vi "kb-Point22.vi"(10 "Src Data":dbl[][](array[numeric]), 11 "ROI Descriptor":T1 {"Contours"."Type" items=["No Selection", "Point", "Line", "Rectangle", "Oval", "Polygon", "Freehand Region", "Annulus", "Unused2", "Unused3", "Broken Line", "Freehand Line", "Rotated Rectangle"]}) -> ()   [LabVIEW 2015]
uses:
  <vilib>/Math Plots/3D Math Plots/3D Surface/3D Surface XCtrl/3D Surface.xctl
  <vilib>/Math Plots/3D Math Plots/3D Surface/3D Surface Datatype/Public/Plot Helper (Matrix).vi
  <vilib>/Math Plots/3D Math Plots/3D Surface/3D Surface Datatype/3D Surface Datatype.lvclass
panel:
  out "3D Surface 3":refnum<class "3D Plot Datatype.lvclass">[](xcontrol) caption="三维曲面"
  out "最大值":dbl
  out "3D Surface 2":refnum<class "3D Plot Datatype.lvclass">[](xcontrol) caption="三维曲面"
  out "3D Surface":refnum<class "3D Plot Datatype.lvclass">[](xcontrol) caption="三维曲面"
  out "Coordinates 2":i32[](array[numeric])
  out "Radius (Pixels)":dbl
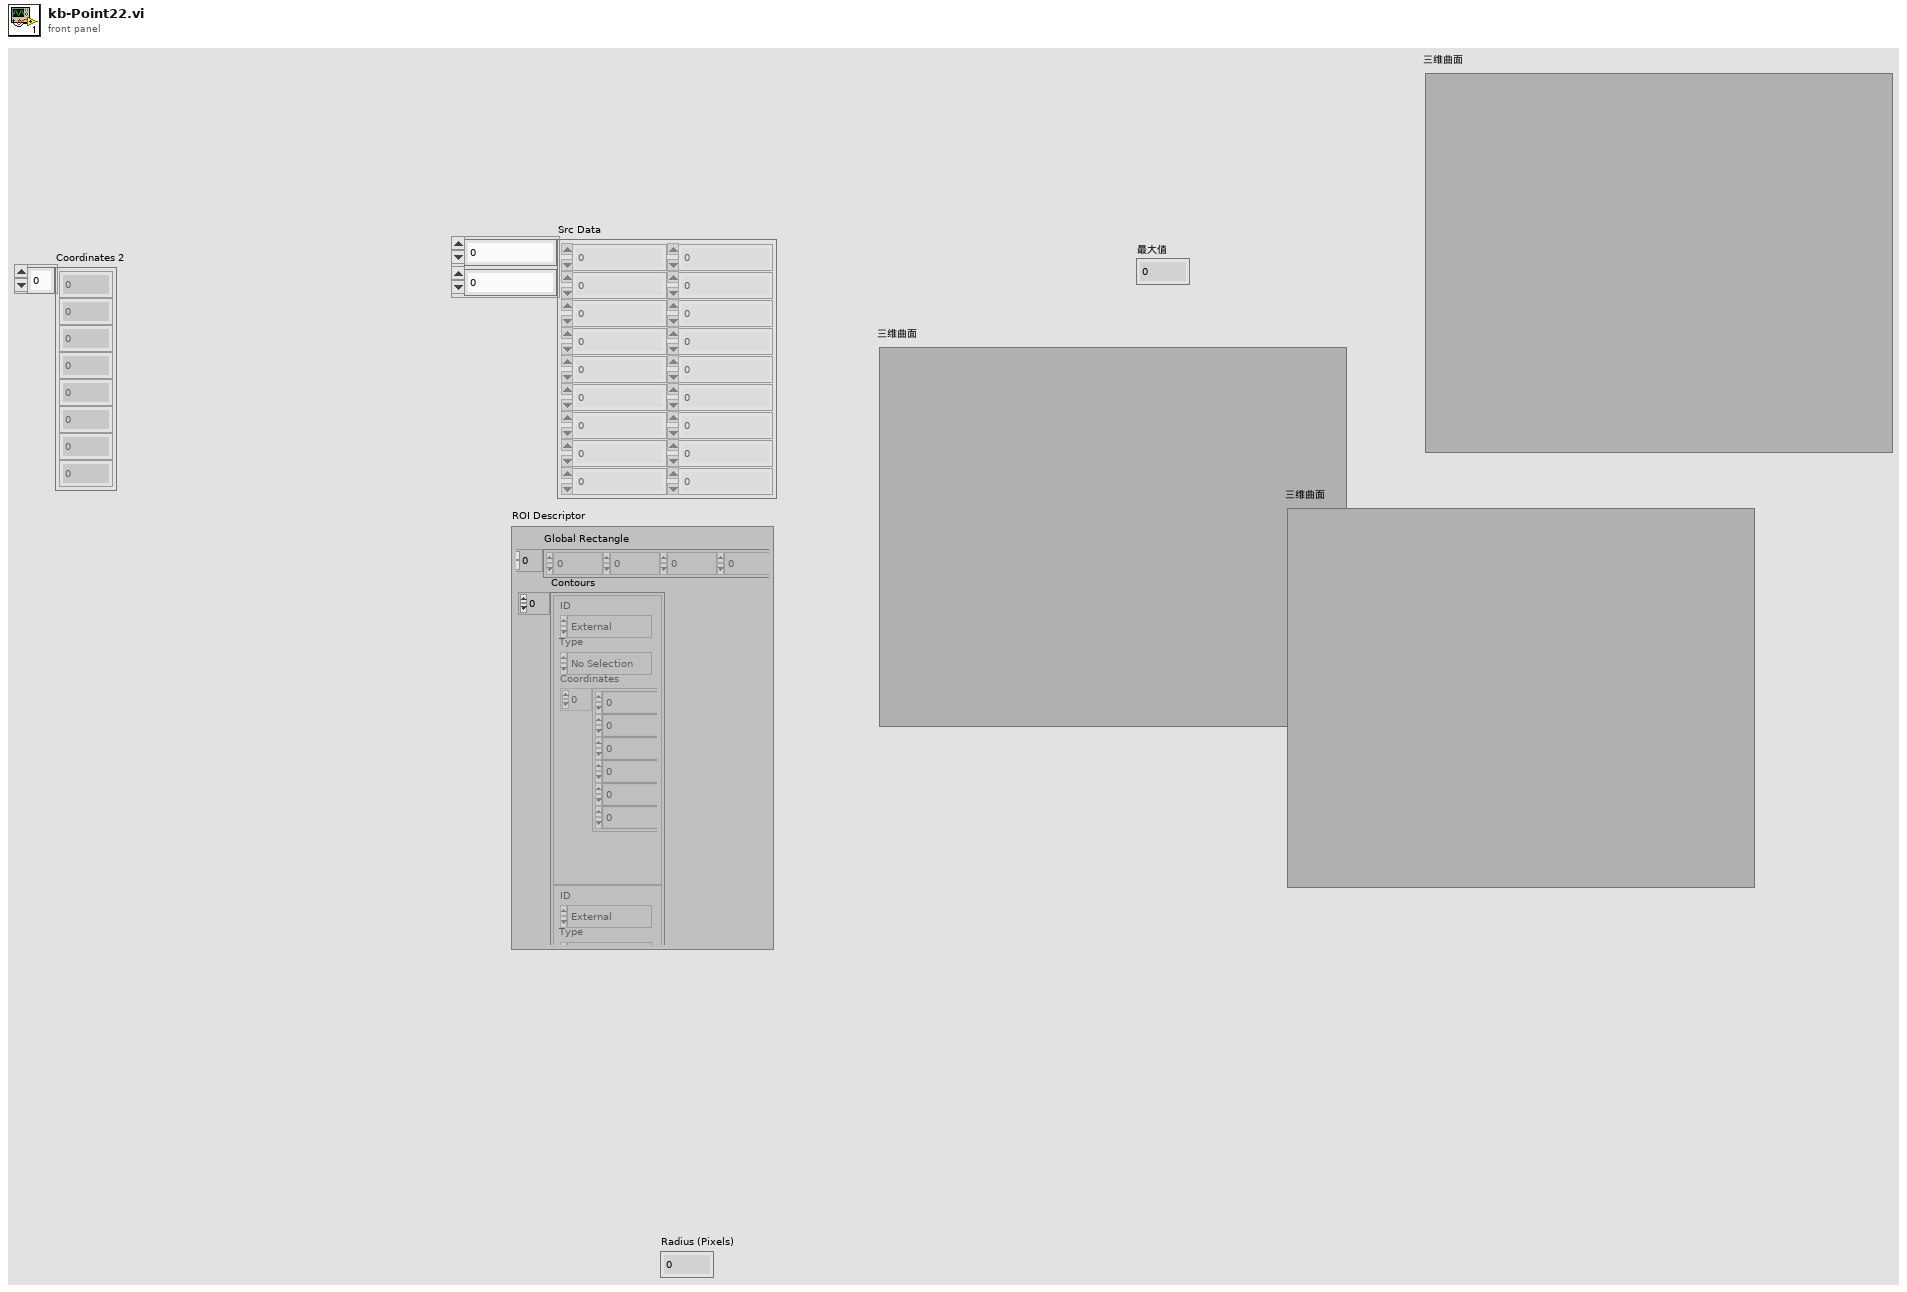
[diagram p1: front panel]
types:
  T1 = typedef "ROI Descriptor" = cluster{"Global Rectangle":i32[], "Contours":cluster{"ID":enum32{"External", "Internal"}, "Type":u32, "Coordinates":i32[]}[]}
  T2 = cluster{"ID":enum32{"External", "Internal"}, "Type":u32, "Coordinates":i32[]}[]
  T3 = cluster{"ID":enum32{"External", "Internal"}, "Type":u32, "Coordinates":i32[]}
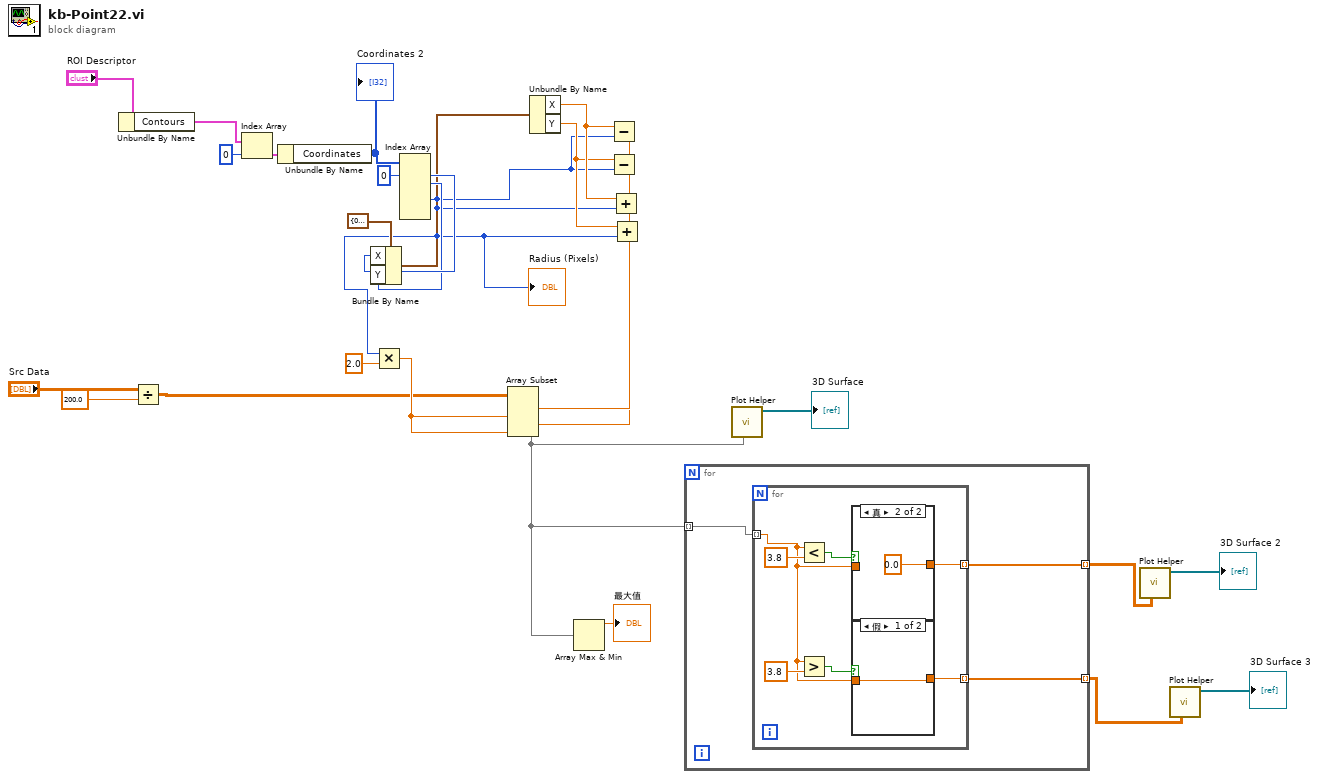
[diagram p0: block diagram]
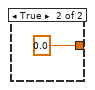
[diagram p2: hidden frame]
diagram:
  n1 = Unbundle By Name("ROI Descriptor") -> ("Contours"=w22:T2)
  n2 = Divide(x="Src Data", y=200.0) -> (x/y=w11:dbl[][])
  n3 = Index Array(array=w22, index=0 ("索引")) -> (element=w20:T3)
  n4 = Unbundle By Name(w20) -> ("Coordinates"=w19:i32[])
  "Coordinates 2" <- w19
  n5 = Index Array(array=w19, index #1=0 ("索引")) -> (element #1=w16:i32, element #2=w15:i32, element #4=w8:i32)  [unwired: 5 in, 3 out]
  "Radius (Pixels)" <- w8
  n6 = Bundle By Name(cluster=cluster{"Y":dbl, "X":dbl} {"Y"=0.0, "X"=0.0}, "X"=w16, "Y"=w15) -> (w14:cluster{"Y":dbl, "X":dbl})
  n7 = Multiply(x=w8, y=2.0) -> (x*y=w24:dbl)
  n8 = Unbundle By Name(w14) -> ("X"=w10:dbl, "Y"=w9:dbl)
  n9 = Subtract(x=w10, y=w8) -> (x-y=w12:dbl)
  n10 = Subtract(x=w9, y=w8) -> (x-y=w23:dbl)
  n11 = Array Subset(array=w11, index (row)=w23, length (row)=w24, index (col)=w12, length (col)=w24) -> (w4:dbl[][])
  n12 = Array Max & Min(array=w4) -> (max value=→"最大值":dbl)  [unwired: 3 out]
  n13 = Add(x=w10, y=w8) -> ()  [unwired: 1 out]
  n14 = Add(x=w9, y=w8) -> ()  [unwired: 1 out]
  n15 = for {
    tunnel: w4 -> [w30] mode=indexing
    tunnel: [w29] -> w5 mode=indexing
    tunnel: [w28] -> w1 mode=indexing
    n16 = for {
      tunnel: w30 -> [w32] mode=indexing
      tunnel: [w35] -> w29 mode=indexing
      tunnel: [w31] -> w28 mode=indexing
      n17 = Less?(x=w32, y=3.8) -> (x < y?=w36:bool)
      n18 = Greater?(x=w32, y=3.8) -> (0:w34:bool)
      n19 = case shown="真" w36 {
        tunnel: [w40 0.0 ("y")] -> w35
        tunnel: w32 -> [w40 _]
        frame False {
        }
        frame True {
        }
      }
      n20 = case shown="假" w34 {
        tunnel: [w38 0.0 ("y")] -> w31
        tunnel: w32 -> [w38 _]
        frame False {
        }
        frame True {
        }
      }
    }
  }
  n21 = call-poly <vilib>:"Plot Helper.vi"("z matrix"=w4) -> ("3D Plot lvclass Array out"=→"3D Surface":refnum<class "3D Plot Datatype.lvclass">[])  [unwired: 5 in, 5 out]
  n22 = call-poly <vilib>:"Plot Helper.vi"("z matrix"=w5) -> ("3D Plot lvclass Array out"=→"3D Surface 2":refnum<class "3D Plot Datatype.lvclass">[])  [unwired: 5 in, 5 out]
  n23 = call-poly <vilib>:"Plot Helper.vi"("z matrix"=w1) -> ("3D Plot lvclass Array out"=→"3D Surface 3":refnum<class "3D Plot Datatype.lvclass">[])  [unwired: 5 in, 5 out]
